vi "Logic_Main.vi"() -> ()   [LabVIEW 2016]
uses:
  Common/public/vis/CMN_FVAR_action.ctl
  private/vis/LOGIC_gbls.vi
  DBSHAND/private/vis/DatabaseHand_Element_Set(string).vi
  DBSHAND/private/vis/DatabaseHand_Element_Set(I32).vi
panel:
  in  "createwhen":string="onreadstart"
  in  "unsctmout":i32=35000
  in  "av_algors":string
  in  "logfile":path=path "/home/arclogs/MOD_LOGIC.log"
  out "ConfigFile":path
  out "stop":bool
  in  "send":bool
  in  "local cmds":string="SHUTDOWN"
  in  "log?":bool
  in  "default algor":string="ccd"
  in  "Config":string[][](table)=[["LOG", "log", "Logic_Main.vi", "log?", "no", "BOOL"], ["LOG", "file", "Logic_Main.vi", "logfile", "", "PATH"], ["ALGORS", "dir", "Logic_Main.vi", "algors dir", "", "PATH"], ["ALGORS", "default", "Logic_Main.vi", "default algor", "ccd", "STR"], ["ALGORS", "logdir", "Logic_Main.vi", "log dir", "", "PATH"], ["ALGORS", "available", "Logic_Main.vi", "av_algors", "", "STR"], ["ALGORS", "unsctmout", "Logic_Main.vi", "unsctmout", "", "I32"], ["ALGORS", "createwhen", "Logic_Main.vi", "createwhen", "", "STR"]]
  in  "log dir":path=path "/home/arclogs"
  in  "algors dir":path=path "/home/ArcVIEW/Modules/Logical/Algors"
  in  "AVAPP Cmd Proc":refnum<vi>
  out "error out":errorcluster
  in  "error in":errorcluster
  in  "Module Name":string="Logical"
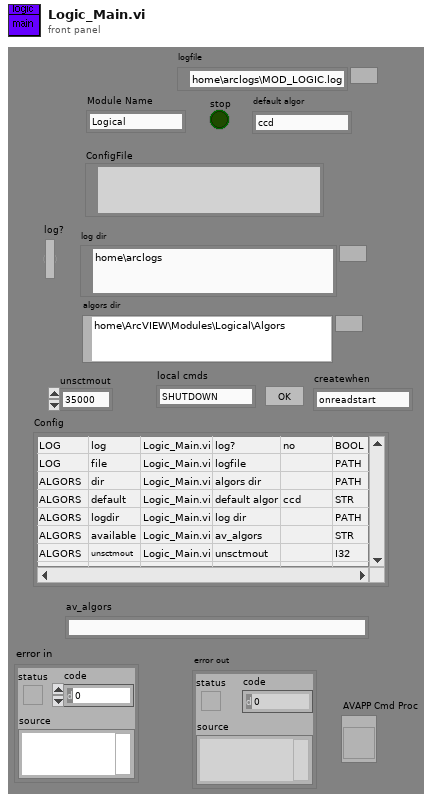
[diagram p1: front panel]
types:
  T1 = typedef "DatabaseHand_RefNum.ctl" = refnum<vi>
  T2 = typedef "CMN_FVAR_action.ctl" = enum16{"read", "write"}
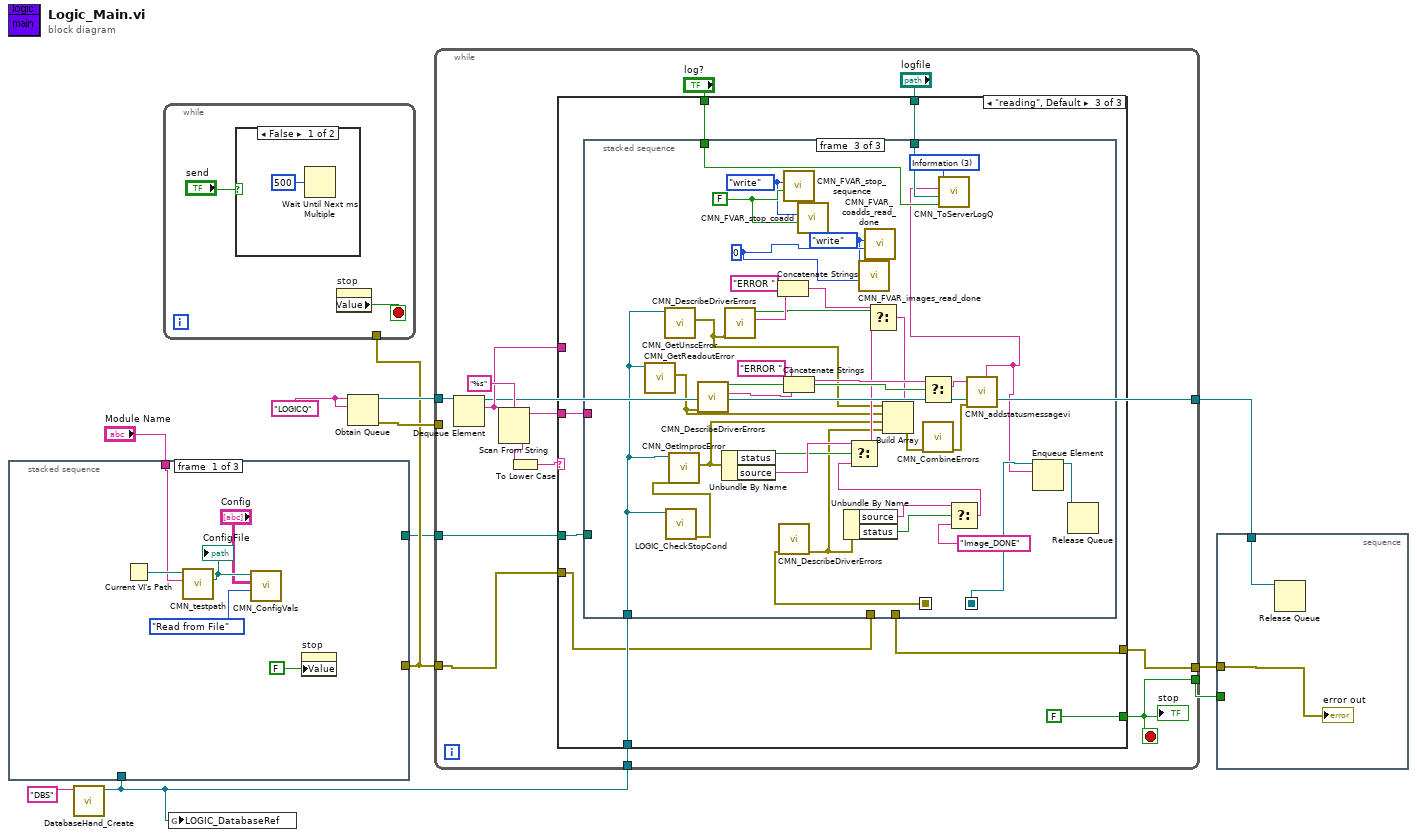
[diagram p0: block diagram]
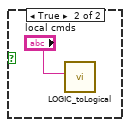
[diagram p2: hidden frame]
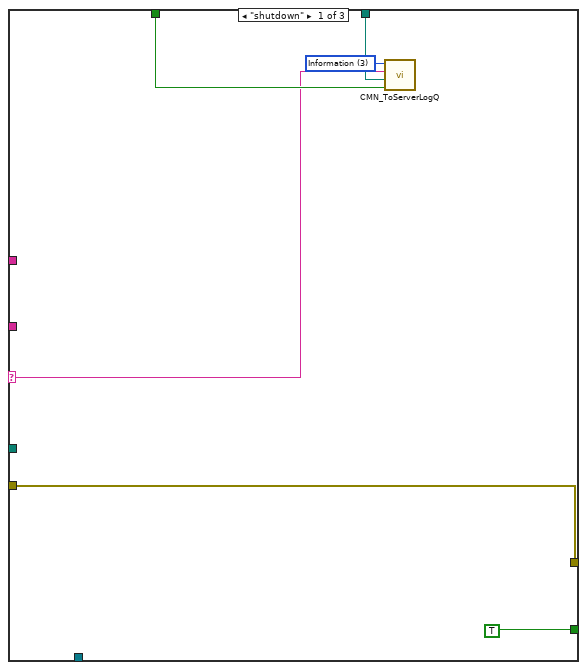
[diagram p3: hidden frame]
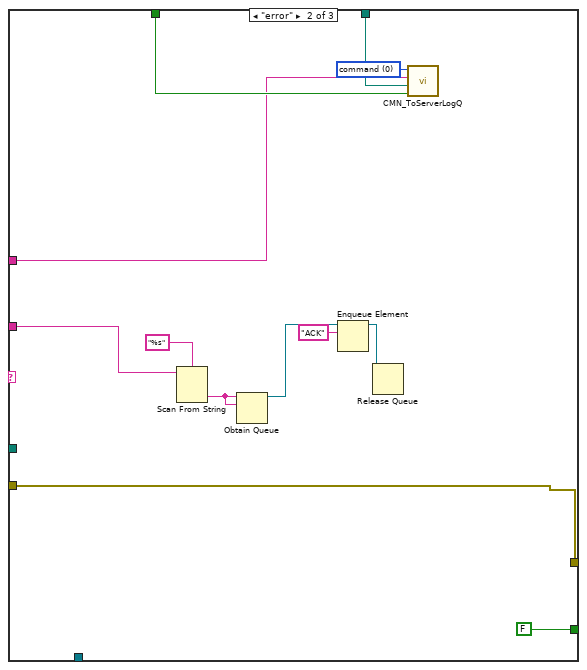
[diagram p4: hidden frame]
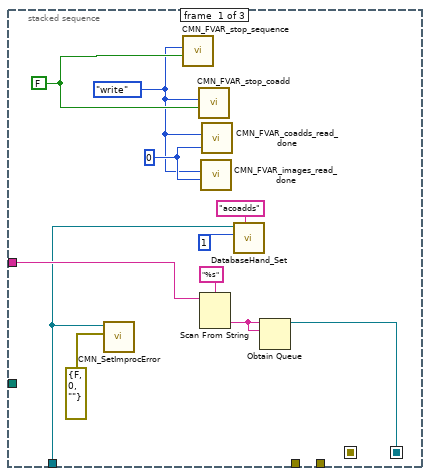
[diagram p5: hidden frame]
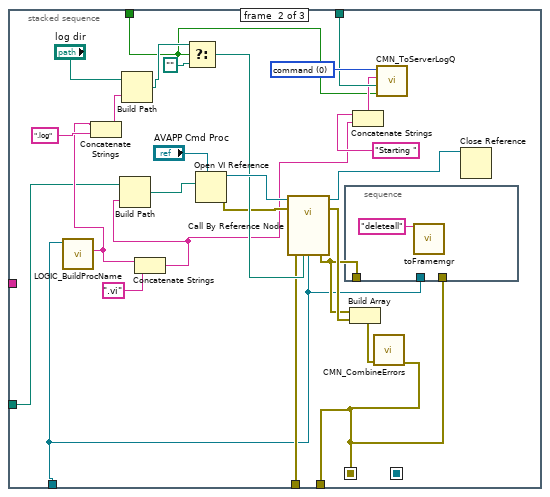
[diagram p6: hidden frame]
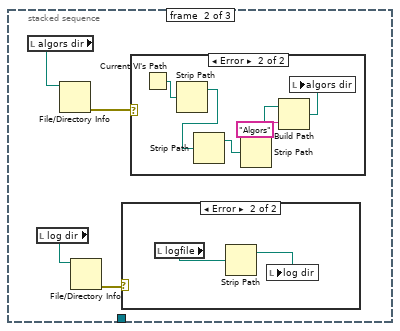
[diagram p7: hidden frame]
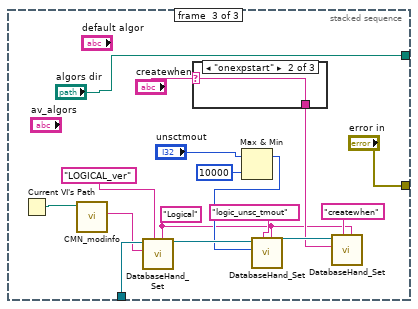
[diagram p10: hidden frame]
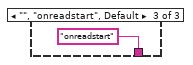
[diagram p12: hidden frame]
diagram:
  w6 = "LOGICQ" ("name (unnamed)")
  n1 = call "DatabaseHand_Create.vi"("Name"="DBS") -> ("Database RefNum out"=w7:T1)  [unwired: 1 in, 9 out]
  n2 = stacked-sequence {
    tunnel: [_ _ "error in"] -> w2
    tunnel: "Module Name" -> [w12 _ _]
    tunnel: w7 -> [_ _ w43]
    tunnel: [_ _ "algors dir"] -> w1
    frame #0 {
      n3 = Current VI's Path() -> (path=w17:path)
      n4 = call "CMN_testpath.vi"("ModuleName"=w12, "caller Path"=w17) -> ("ConfigFile"=w16:path)  [unwired: 1 in, 8 out]
      "ConfigFile" <- w16
      n5 = call "CMN_ConfigVals.vi"("Action"=enum16{"Read from File", "Write to File"}."Read from File", "ConfigVariables"="Config", "configuration file path"=w16) -> ()  [unwired: 1 in, 8 out]
      n6 = property on="stop" class="Bool (strict)"("Value"=FALSE ("stop")) -> ()  [unwired: 2 in, 2 out]
    }
    frame #1 {
      n7 = local read "algors dir"() -> (w19:path)
      n8 = local read "log dir"() -> (w21:path)
      n9 = File/Directory Info(path=w19) -> (error out=w18:errorcluster)  [unwired: 1 in, 6 out]
      n10 = File/Directory Info(path=w21) -> (error out=w20:errorcluster)  [unwired: 1 in, 6 out]
      n11 = case shown="Error" w20 {
        frame No Error {
        }
        frame Error {
          n12 = local read "logfile"() -> (w29:path)
          n13 = Strip Path(path=w29) -> (stripped path=w28:path)  [unwired: 1 out]
          n14 = local write "log dir"(w28) -> ()
        }
      }
      n15 = case shown="Error" w18 {
        frame No Error {
        }
        frame Error {
          n16 = Current VI's Path() -> (path=w27:path)
          n17 = Strip Path(path=w27) -> (stripped path=w24:path)  [unwired: 1 out]
          n18 = Strip Path(path=w24) -> (stripped path=w23:path)  [unwired: 1 out]
          n19 = Strip Path(path=w23) -> (stripped path=w22:path)  [unwired: 1 out]
          n20 = Build Path(base path=w22, name or relative path="Algors") -> (appended path=w25:path)
          n21 = local write "algors dir"(w25) -> ()
        }
      }
    }
    frame #2 {
      w30 = "Logical" ("group")
      n22 = Current VI's Path() -> (path=w44:path)
      n23 = call "CMN_modinfo.vi"("caller path"=w44) -> ("INFO"=w42:string)  [unwired: 2 in, 8 out]
      n24 = call-poly "DatabaseHand_Set.vi"("group"=w30, "name"="LOGICAL_ver", "value"=w42, "Database RefNum in"=w43) -> ("Database RefNum out"=w39:T1)  [unwired: 4 in, 3 out]
      n25 = case shown="\"onexpstart\"" "createwhen" {
        selector: "createwhen" -> [w46 w47 _]
        tunnel: [w46 w47 "onreadstart" ("createwhen")] -> w31
        frame "onreadend" {
        }
        frame "onexpstart" {
        }
        frame "", "onreadstart", Default {
        }
      }
      n26 = Max & Min(x="unsctmout", y=10000) -> (max(x,y)=w35:i32)  [unwired: 1 out]
      n27 = call-poly "DatabaseHand_Set.vi"("group"=w30, "name"="logic_unsc_tmout", "value"=w35, "Database RefNum in"=w39) -> ("Database RefNum out"=w34:T1)  [unwired: 4 in, 3 out]
      n28 = call-poly "DatabaseHand_Set.vi"("group"=w30, "name"="createwhen", "value"=w31, "Database RefNum in"=w34) -> ()  [unwired: 4 in, 4 out]
    }
  }
  n29 = while {
    tunnel: w2 -> [_]
    stop <- w50 stop-if-true
    n30 = case shown="False" "send" {
      frame False {
        n31 = Wait Until Next ms Multiple(millisecond multiple=u32 500) -> ()  [unwired: 1 out]
      }
      frame True {
        n32 = call "LOGIC_toLogical.vi"("command"="local cmds") -> ()  [unwired: 1 in, 9 out]
      }
    }
    n33 = property on="stop" class="Bool (strict)"() -> ("Value"=w50:bool)  [unwired: 2 in, 2 out]
  }
  n34 = global write "LOGIC_gbls.vi" "LOGIC_DatabaseRef"(w7) -> ()
  n35 = Obtain Queue(name (unnamed)=w6, element data type=w6) -> (queue out=w5:refnum<queue>, error out=w4:errorcluster)  [unwired: 3 in, 1 out]
  n36 = while {
    tunnel: [w64] -> w10
    tunnel: w2 -> [w65]
    tunnel: [w66] -> w11
    tunnel: w4 -> [_]
    tunnel: w7 -> [w57]
    tunnel: w5 -> [w56]
    tunnel: [w54] -> w3
    tunnel: w1 -> [w53]
    stop <- w66 stop-if-true
    n37 = Dequeue Element(queue=w56) -> (queue out=w54:refnum<queue>, element=w55:string)  [unwired: 1 in, 3 out]
    n38 = Scan From String(format string="%s", input string=w55) -> (remaining string=w60:string, output 1=w62:string)  [unwired: 2 in, 3 out]
    n39 = To Lower Case(string=w62) -> (all lower case string=w61:string)
    n40 = case shown="\"reading\", Default" w61 {
      selector: w61 -> [w68 _ _]
      tunnel: [TRUE FALSE FALSE] -> w66
      tunnel: w65 -> [w71 w84 w87]
      tunnel: [w71 w84 w91] -> w64
      tunnel: w60 -> [_ w74 w86]
      tunnel: "log?" -> [w69 w80 w90]
      tunnel: "logfile" -> [w70 w82 w89]
      tunnel: w57 -> [_ _ w88]
      tunnel: w55 -> [_ w73 _]
      tunnel: w53 -> [_ _ w85]
      frame "shutdown" {
        w67 = u16 3 items=["command", "imediateReply", "Callback Reply", "Information"] ("type")
        (unwired) TRUE
        n41 = call "CMN_ToServerLogQ.vi"("Log"=w69, "file"=w70, "string"=w68, "type"=w67) -> ()  [unwired: 2 in, 5 out]
      }
      frame "error" {
        w81 = u16 0 items=["command", "imediateReply", "Callback Reply", "Information"] ("type")
        n42 = Scan From String(format string="%s", input string=w74) -> (output 1=w77:string)  [unwired: 2 in, 4 out]
        n43 = Obtain Queue(name (unnamed)=w77, element data type=w77) -> (queue out=w76:refnum<queue>)  [unwired: 3 in, 2 out]
        n44 = Enqueue Element(queue=w76, element="ACK") -> (queue out=w79:refnum<queue>)  [unwired: 1 in, 3 out]
        n45 = Release Queue(queue=w79) -> ()  [unwired: 1 in, 4 out]
        n46 = call "CMN_ToServerLogQ.vi"("Log"=w80, "file"=w82, "string"=w73, "type"=w81) -> ()  [unwired: 2 in, 5 out]
      }
      frame "reading", Default {
        (unwired) FALSE
        n47 = stacked-sequence {
          seq-local: [_ w104 _] -> [_ _ w133]
          seq-local: [w99 _ _] -> [_ _ w148]
          tunnel: [_ w104 _] -> w91
          tunnel: w89 -> [_ w119 w151]
          tunnel: w90 -> [_ w116 w150]
          tunnel: w88 -> [w94 w110 w145]
          tunnel: w87 -> [_ w115 _]
          tunnel: w86 -> [w102 _ _]
          tunnel: w85 -> [_ w107 _]
          frame #0 {
            w93 = CMN_FVAR_action."write" ("action")
            w95 = u16 0 ("coadds done")
            w96 = FALSE ("Sequence was Stoped")
            n48 = call "CMN_SetImprocError.vi"("improc error"=errorcluster {"status"=FALSE, "code"=0, "source"=""} ("picread Error"), "Database RefNum in"=w94) -> ()  [unwired: 1 in, 9 out]
            n49 = call "CMN_FVAR_stop_sequence.vi"("value in"=w96, "action"=w93) -> ()  [unwired: 9 out]
            n50 = call "CMN_FVAR_stop_coadd.vi"("value in"=w96, "action"=w93) -> ()  [unwired: 9 out]
            n51 = Scan From String(format string="%s", input string=w102) -> (output 1=w100:string)  [unwired: 2 in, 4 out]
            n52 = call "CMN_FVAR_images_read_done.vi"("value in"=w95, "action"=w93) -> ()  [unwired: 9 out]
            n53 = call "CMN_FVAR_coadds_read_done.vi"("value in"=w95, "action"=w93) -> ()  [unwired: 9 out]
            n54 = call-poly "DatabaseHand_Set.vi"("name"="acoadds", "value"=1, "Database RefNum in"=w94) -> ()  [unwired: 5 in, 4 out]
            n55 = Obtain Queue(name (unnamed)=w100, element data type=w100) -> (queue out=w99:refnum<queue>)  [unwired: 3 in, 2 out]
          }
          frame #1 {
            w120 = u16 0 items=["command", "imediateReply", "Callback Reply", "Information"] ("type")
            n56 = call "LOGIC_BuildProcName.vi"("Database RefNum in"=w110) -> ("proc name"=w109:string)  [unwired: 10 out]
            n57 = Concatenate Strings(w109, ".log" ("string")) -> (w124:string)
            n58 = Build Path(base path="log dir", name or relative path=w124) -> (appended path=w122:path)
            n59 = Concatenate Strings(w109, ".vi") -> (w105:string)
            n60 = Build Path(base path=w107, name or relative path=w105) -> (appended path=w106:path)
            n61 = Select(t=w122, s=w116, f=path "") -> (s? t:f=w121:path)
            n62 = Open VI Reference(type specifier VI Refnum (for type only)="AVAPP Cmd Proc", vi path=w106) -> (vi reference=w128:refnum<vi>, error out=w114:errorcluster)  [unwired: 1 in, 3 out]
            n63 = call-by-ref "Call By Reference Node"(reference=w128, error in=w114, 11:"error in (no error)"=w115, "logfile"=w121, "Database RefNum out"=w110) -> (reference out=w108:refnum<vi>, error out=w113:errorcluster, 15:"error out"=w111:errorcluster)  [unwired: 12 in]
            n64 = Build Array(w111, w113) -> (w112:errorcluster[])
            n65 = Concatenate Strings("Starting " ("string"), w105) -> (w117:string)
            n66 = call "CMN_CombineErrors.vi"("Errors"=w112) -> ("error out"=w104:errorcluster)  [unwired: 10 out]
            n67 = stacked-sequence {
              tunnel: w111 -> [_]
              tunnel: w110 -> [_]
              tunnel: w104 -> [_]
              frame #0 {
                n68 = call "toFramemgr.vi"("command"="deleteall") -> ()  [unwired: 8 in, 7 out]
              }
            }
            n69 = call "CMN_ToServerLogQ.vi"("Log"=w116, "file"=w119, "string"=w117, "type"=w120) -> ()  [unwired: 2 in, 5 out]
            n70 = Close Reference(reference=w108) -> ()  [unwired: 1 in, 1 out]
          }
          frame #2 {
            w140 = CMN_FVAR_action."write" ("action")
            w142 = CMN_FVAR_action."write" ("action")
            w149 = u16 3 items=["command", "imediateReply", "Callback Reply", "Information"] ("type")
            w141 = u16 0 ("coadds done")
            w143 = FALSE ("Sequence was Stoped")
            n71 = call "CMN_GetReadoutError.vi"("Database RefNum in"=w145) -> ("readout_error"=w138:errorcluster)  [unwired: 1 in, 9 out]
            n72 = call "CMN_GetUnscError.vi"("Database RefNum in"=w145) -> ("unsc_error"=w139:errorcluster)  [unwired: 1 in, 9 out]
            n73 = call "LOGIC_CheckStopCond.vi"("Database RefNum in"=w145) -> ("error out"=w144:errorcluster)  [unwired: 1 in, 9 out]
            n74 = call "CMN_GetImprocError.vi"("error in (no error)"=w144, "Database RefNum in"=w145) -> ("improc_error"=w137:errorcluster)  [unwired: 9 out]
            n75 = call "CMN_DescribeDriverErrors.vi"("error in (no error)"=w138) -> ("error?"=w163:bool, "astroerrors"=w164:string)  [unwired: 4 in, 4 out]
            n76 = Unbundle By Name(w137) -> ("status"=w165:bool, "source"=w166:string)
            n77 = call "CMN_DescribeDriverErrors.vi"("error in (no error)"=w139) -> ("error?"=w159:bool, "astroerrors"=w160:string)  [unwired: 4 in, 4 out]
            n78 = Concatenate Strings("ERROR ", w160) -> (w158:string)
            n79 = call "CMN_DescribeDriverErrors.vi"("error in (no error)"=w133) -> ("error out"=w132:errorcluster)  [unwired: 4 in, 5 out]
            n80 = call "CMN_FVAR_stop_sequence.vi"("value in"=w143, "action"=w142) -> ()  [unwired: 9 out]
            n81 = Concatenate Strings("ERROR ", w164) -> (w162:string)
            n82 = call "CMN_FVAR_stop_coadd.vi"("value in"=w143, "action"=w142) -> ()  [unwired: 9 out]
            n83 = Unbundle By Name(w132) -> ("source"=w134:string, "status"=w156:bool)
            n84 = call "CMN_FVAR_images_read_done.vi"("value in"=w141, "action"=w140) -> ()  [unwired: 9 out]
            n85 = call "CMN_FVAR_coadds_read_done.vi"("value in"=w141, "action"=w140) -> ()  [unwired: 9 out]
            n86 = Build Array(w139, w138, w137, w132) -> (w136:errorcluster[])
            n87 = call "CMN_CombineErrors.vi"("Errors"=w136) -> ("error out"=w135:errorcluster)  [unwired: 10 out]
            n88 = Select(t=w134, s=w156, f="Image_DONE") -> (s? t:f=w153:string)
            n89 = Select(t=w166, s=w165, f=w153) -> (s? t:f=w154:string)
            n90 = Select(t=w158, s=w159, f=w154) -> (s? t:f=w155:string)
            n91 = Select(t=w162, s=w163, f=w155) -> (s? t:f=w146:string)
            n92 = call "CMN_addstatusmessagevi.vi"("error in (no error)"=w135, "message  in"=w146) -> ("modified message out"=w131:string)  [unwired: 9 out]
            n93 = call "CMN_ToServerLogQ.vi"("Log"=w150, "file"=w151, "string"=w131, "type"=w149) -> ()  [unwired: 2 in, 5 out]
            n94 = Enqueue Element(queue=w148, element=w131) -> (queue out=w147:refnum<queue>)  [unwired: 1 in, 3 out]
            n95 = Release Queue(queue=w147) -> ()  [unwired: 1 in, 4 out]
          }
        }
      }
    }
    "stop" <- w66
  }
  n96 = stacked-sequence {
    tunnel: w11 -> [_]
    tunnel: w10 -> [w168]
    tunnel: w3 -> [w167]
    frame #0 {
      n97 = Release Queue(queue=w167) -> ()  [unwired: 1 in, 4 out]
      "error out" <- w168
    }
  }
